vi "shortcut_keys.vi"() -> ()   [LabVIEW 2023]
panel:
  in  "ショートカットキー 13":bool
  in  "ショートカットキー 12":bool
  in  "ショートカットキー 11":bool
  in  "ショートカットキー 10":bool
  in  "ショートカットキー 9":bool
  in  "ショートカットキー 8":bool
  in  "ショートカットキー 7":bool
  in  "ショートカットキー 6":bool
  in  "ショートカットキー 5":bool
  in  "ショートカットキー 4":bool
  in  "ショートカットキー 3":bool
  in  "ショートカットキー 2":bool
  in  "ショートカットキー":bool
  in  "ループ時間設定（ｍS）":u32
  in  "2.Switch when released（離したときに切り替え）":bool
  out "Boolean 6":bool
  out "Boolean 5":bool
  out "Boolean 4":bool
  out "Boolean 3":bool
  out "Boolean 2":bool
  out "Boolean":bool
  in  "6.Latch until released（3+5のラッチ）":bool
  in  "5.Latch when released（離したときにラッチ）":bool
  in  "4.Latch when pressed（押したときにラッチ）":bool
  in  "3.Switch until released（押している間だけ切り替え）":bool
  in  "stop":bool
  in  "1.Switch when pressed（押したときに切り替え）":bool
  # "スイッチ操作6種"
  # "スイッチ操作は６種類の動作を設定できます\n設定は、プロパティ内Operationもしくは右クリックMechanicalActionで行います。"
  # "ボタンが押されると状態が切り替わり、その状態を維持します。再度ボタンを押すまでその状態は変わりません。\nロック式スイッチの動作"
  # "ボタンを押したあと離した状態になったときに切り替わり、その状態を保持します。\n再度ボタンを押して離すまで、状態は変わりません。"
  # "ボタンを押している間だけ状態が変わり、離すと元の状態に戻ります。\n押している間だけ一時的に状態が変わる動作です。モーメンタリースイッチの動作"
  # "ボタンを押すとワンショットパルス(True)が出ます。"
  # "⇒⇒⇒"
  # "※スイッチ動作は4.Latch when pressedに設定"
  # "ボタンを押したあと離した状態になったときにワンショットパルス（True）が出ます。"
  # "・・・・・・・・・・・・"
  # "ボタンを押しはじめから離したあとしばらくTrueな状態になります\n３と５の動作が合わさった動きです。"
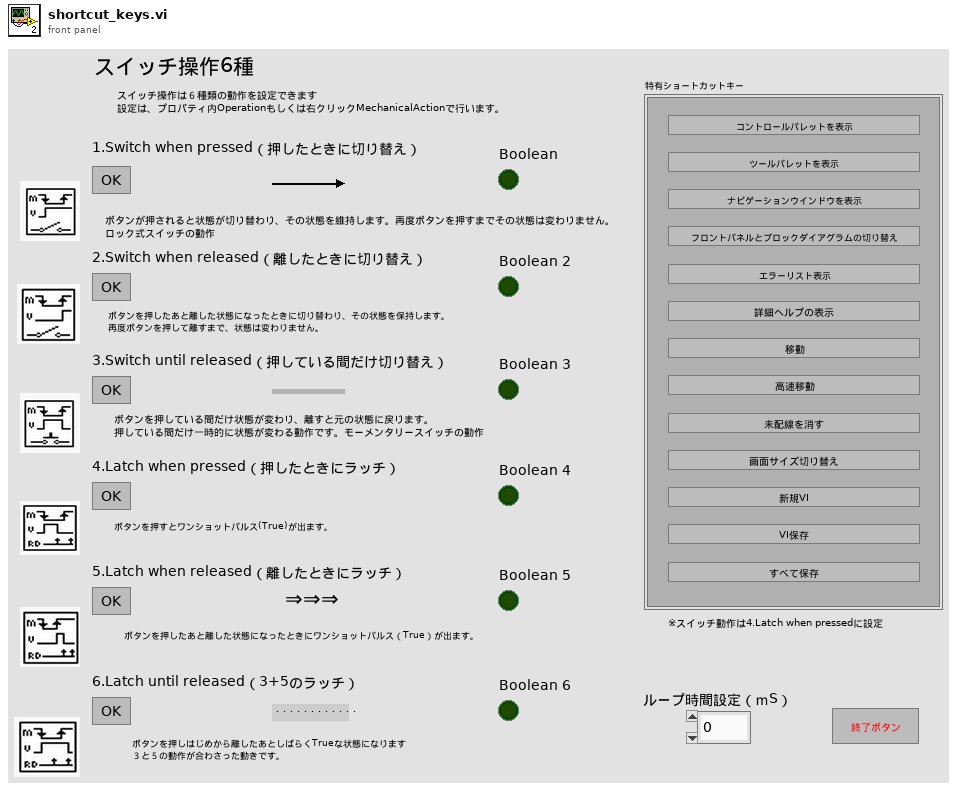
[diagram p1: front panel]
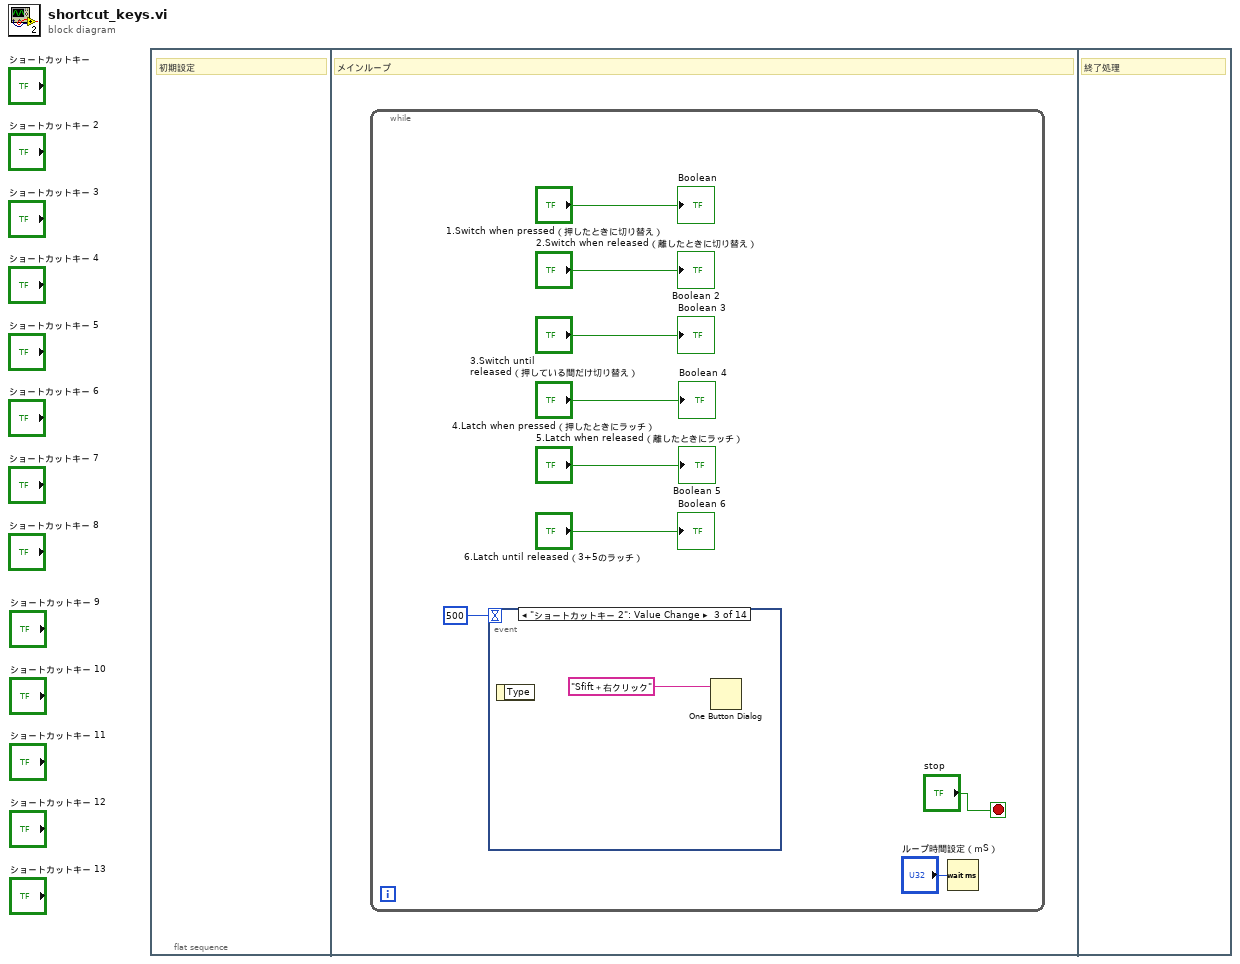
[diagram p0: block diagram]
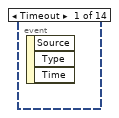
[diagram p2: hidden frame]
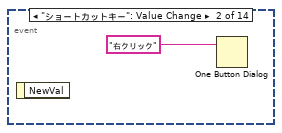
[diagram p3: hidden frame]
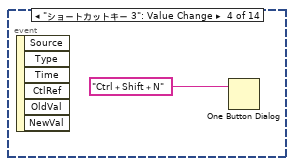
[diagram p4: hidden frame]
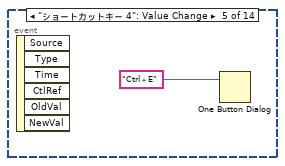
[diagram p5: hidden frame]
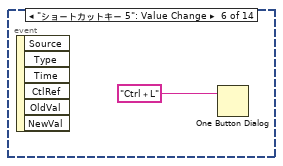
[diagram p6: hidden frame]
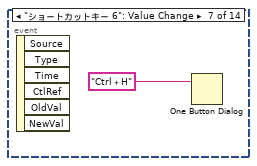
[diagram p7: hidden frame]
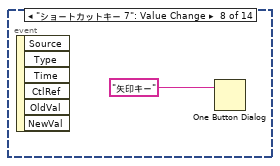
[diagram p8: hidden frame]
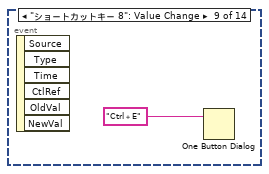
[diagram p9: hidden frame]
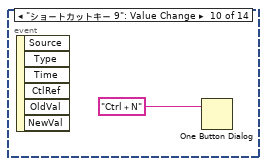
[diagram p10: hidden frame]
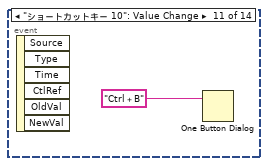
[diagram p11: hidden frame]
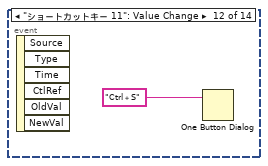
[diagram p12: hidden frame]
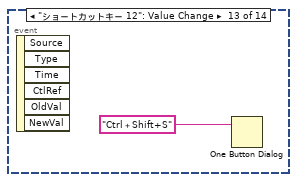
[diagram p13: hidden frame]
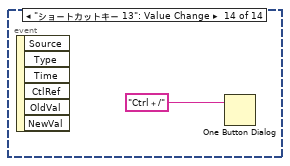
[diagram p14: hidden frame]
diagram:
  n1 = flat-sequence {
    frame #0 {
      # "初期設定"
    }
    frame #1 {
      # "メインループ"
      n2 = while {
        stop <- "stop" stop-if-true
        n3 = event shown="[2] \"ショートカットキー 2\": Value Change" {
          selector: _ -> [_ _ _ _ _ _ _ _ _ _ _ _ _ _]
          dyn-events: _ -> [_ _ _ _ _ _ _ _ _ _ _ _ _ _]
          timeout: 500 -> [_ _ _ _ _ _ _ _ _ _ _ _ _ _]
          event Timeout {
            n4 = event-data() -> ()  [unwired: 1 in, 3 out]
          }
          event "ショートカットキー": Value Change {
            n5 = event-data() -> ()  [unwired: 1 in, 1 out]
            n6 = One Button Dialog(message="右クリック") -> ()  [unwired: 1 in, 1 out]
          }
          event "ショートカットキー 2": Value Change {
            n7 = event-data() -> ()  [unwired: 1 in, 1 out]
            n8 = One Button Dialog(message="Sfift＋右クリック") -> ()  [unwired: 1 in, 1 out]
          }
          event "ショートカットキー 3": Value Change {
            n9 = event-data() -> ()  [unwired: 1 in, 6 out]
            n10 = One Button Dialog(message="Ctrl＋Shift＋N") -> ()  [unwired: 1 in, 1 out]
          }
          event "ショートカットキー 4": Value Change {
            n11 = event-data() -> ()  [unwired: 1 in, 6 out]
            n12 = One Button Dialog(message="Ctrl＋E") -> ()  [unwired: 1 in, 1 out]
          }
          event "ショートカットキー 5": Value Change {
            n13 = event-data() -> ()  [unwired: 1 in, 6 out]
            n14 = One Button Dialog(message="Ctrl＋L") -> ()  [unwired: 1 in, 1 out]
          }
          event "ショートカットキー 6": Value Change {
            n15 = event-data() -> ()  [unwired: 1 in, 6 out]
            n16 = One Button Dialog(message="Ctrl＋H") -> ()  [unwired: 1 in, 1 out]
          }
          event "ショートカットキー 7": Value Change {
            n17 = event-data() -> ()  [unwired: 1 in, 6 out]
            n18 = One Button Dialog(message="矢印キー") -> ()  [unwired: 1 in, 1 out]
          }
          event "ショートカットキー 8": Value Change {
            n19 = event-data() -> ()  [unwired: 1 in, 6 out]
            n20 = One Button Dialog(message="Ctrl＋E") -> ()  [unwired: 1 in, 1 out]
          }
          event "ショートカットキー 9": Value Change {
            n21 = event-data() -> ()  [unwired: 1 in, 6 out]
            n22 = One Button Dialog(message="Ctrl＋N") -> ()  [unwired: 1 in, 1 out]
          }
          event "ショートカットキー 10": Value Change {
            n23 = event-data() -> ()  [unwired: 1 in, 6 out]
            n24 = One Button Dialog(message="Ctrl＋B") -> ()  [unwired: 1 in, 1 out]
          }
          event "ショートカットキー 11": Value Change {
            n25 = event-data() -> ()  [unwired: 1 in, 6 out]
            n26 = One Button Dialog(message="Ctrl＋S") -> ()  [unwired: 1 in, 1 out]
          }
          event "ショートカットキー 12": Value Change {
            n27 = event-data() -> ()  [unwired: 1 in, 6 out]
            n28 = One Button Dialog(message="Ctrl＋Shift+S") -> ()  [unwired: 1 in, 1 out]
          }
          event "ショートカットキー 13": Value Change {
            n29 = event-data() -> ()  [unwired: 1 in, 6 out]
            n30 = One Button Dialog(message="Ctrl＋/") -> ()  [unwired: 1 in, 1 out]
          }
        }
        n31 = Wait (ms)(milliseconds to wait="ループ時間設定（ｍS）") -> ()  [unwired: 1 out]
        "Boolean" <- "1.Switch when pressed（押したときに切り替え）"
        "Boolean 2" <- "2.Switch when released（離したときに切り替え）"
        "Boolean 3" <- "3.Switch until released（押している間だけ切り替え）"
        "Boolean 4" <- "4.Latch when pressed（押したときにラッチ）"
        "Boolean 5" <- "5.Latch when released（離したときにラッチ）"
        "Boolean 6" <- "6.Latch until released（3+5のラッチ）"
      }
    }
    frame #2 {
      # "終了処理"
    }
  }
